vi "Set Initialization Data - TCP Receive.vi"(8 "error in":errorcluster, 11 "Network End Point in":refnum<class "Network End Point.lvclass">) -> (0 "error out":errorcluster, 3 "Network End Point out":refnum<class "Network End Point.lvclass">)   [LabVIEW 2020, in "Network End Point.lvclass"]
doc: "Sets the initialization data of a statically linked subWorker."
uses:
  Network End Point.lvclass
  C:/Program Files (x86)/National Instruments/LabVIEW 2020/vi.lib/addons/_Workers/Library/Classes/Worker/Worker.lvclass
  TCP Receive/Initialization Data.ctl
  <vilib>/addons/_Workers/Library/Classes/Message Queue/Message Queue.lvclass
  <vilib>/addons/_Workers/Library/Classes/Worker/Worker.lvclass/Worker.ctl
  Network End Point.lvclass/Network End Point.ctl
  TCP Receive/TCP Receive.lvclass
  <vilib>/addons/_Workers/Library/Classes/Worker/Worker.lvclass
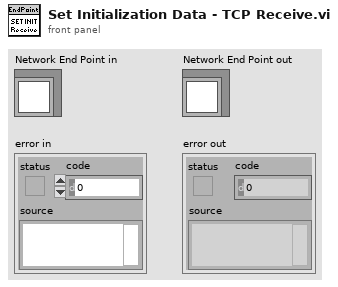
[diagram p1: front panel]
types:
  T1 = typedef "TCP Receive.lvclass/Initialization Data.ctl" = cluster{"String":string, "connection ID":refnum<k5>, "End Point":refnum<class "Message Queue.lvclass">}
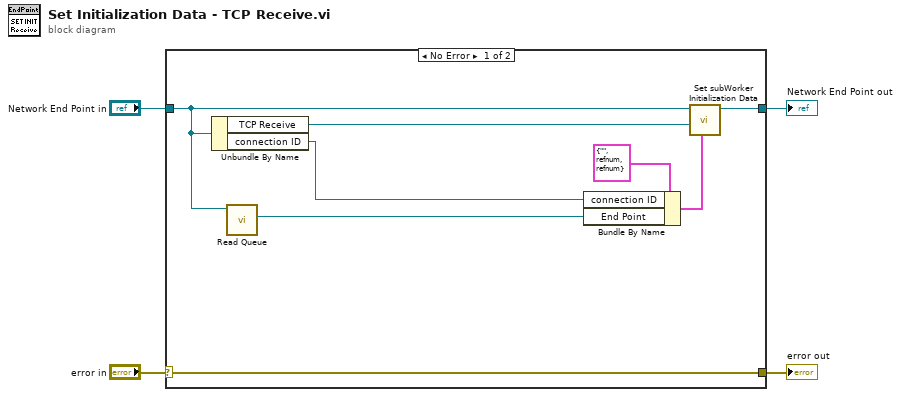
[diagram p0: block diagram]
diagram:
  n1 = case shown="No Error" "error in" {
    selector: "error in" -> [w12 w14]
    tunnel: [w12 w14] -> w3
    tunnel: [w10 w13] -> w2
    tunnel: "Network End Point in" -> [w6 w13]
    frame No Error {
      n2 = Unbundle By Name(w6) -> ("TCP Receive"=w11:refnum<class "TCP Receive.lvclass">, "connection ID"=w7:refnum<k5>)
      n3 = call <vilib>:"Read Queue.vi"("Worker"=w6) -> ("Message Queue out"=w5:refnum<class "Message Queue.lvclass">)  [unwired: 9 in, 1 out]
      n4 = Bundle By Name(cluster=T1 {"String"="", "connection ID"=refnum, "End Point"=refnum} ("Initialization Data"), "connection ID"=w7, "End Point"=w5) -> (w8:T1)
      n5 = call <vilib>:"Set subWorker Initialization Data.vi"("Initialization Data"=w8, "subWorker"=w11, "Worker"=w6) -> ("Worker out"=w10:refnum<class "Network End Point.lvclass">)  [unwired: 8 in]
    }
    frame Error {
    }
  }
  "error out" <- w3
  "Network End Point out" <- w2
